vi "Comulative wheels angles.vi"() -> ()   [LabVIEW 2018]
panel:
  out "back-right":i32
  out "back-left":i32
  out "front-left":i32
  out "front-right":i32
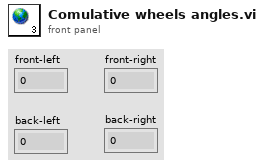
[diagram p1: front panel]
diagram:
